vi "Lab Panel V4.87.vi"() -> ()   [LabVIEW 2013] (continued)
                                n557 = Unbundle(w898) -> ("Tmp Live"=w900:dbl, "Tmp Neut"=w899:dbl)  [unwired: 3 out]
                                n558 = Bundle(cluster=w902, "TL"=w900, "TN"=w899) -> (w901:cluster{"TL":dbl, "TN":dbl})
                                n559 = local write "TEMP START LAB01-2"(w901) -> ()
                              }
                            }
                          }
                        }
                      }
                    }
                  }
                }
              }
              event "RUN LAB02-1": Value Change {
                n560 = event-data() -> ("NewVal"=w907:bool)  [unwired: 1 in, 5 out]
                n561 = local read "SIG LAB02-1"() -> (w903:T2)
                n562 = case shown="True" w907 {
                  tunnel: w913 -> [_ w950]
                  tunnel: w912 -> [_ w949]
                  tunnel: w910 -> [w915 w948]
                  tunnel: w911 -> [_ w947]
                  tunnel: w909 -> [_ w946]
                  tunnel: [w914 w945] -> w908
                  tunnel: w906 -> [_ w944]
                  tunnel: w905 -> [_ w943]
                  tunnel: w904 -> [_ w942]
                  tunnel: w903 -> [_ w941]
                  frame False {
                    # "stop test"
                    n563 = stacked-sequence {
                      tunnel: w915 -> [w924 _]
                      tunnel: [w916 _] -> w914
                      frame #0 {
                        n564 = local read "DISP LAB02-1"() -> (w923:T4)
                        n565 = Unbundle(w923) -> ("CYCLE"=w921:dbl, "MINS"=w922:dbl)  [unwired: 1 out]
                        n566 = case shown="\"CYCLE TEST\"" w924 {
                          tunnel: w922 -> [_ _ w931]
                          tunnel: w921 -> [w929 w930 _]
                          tunnel: [w929 w930 w931] -> w920
                          frame "CHART TEST", Default {
                          }
                          frame "CYCLE TEST" {
                          }
                          frame "T-RISE TEST" {
                          }
                        }
                        n567 = local read "TDMS LAB02-1"() -> (w928:refnum<k34>)
                        n568 = Build Array("STOPPED") -> (w925:string[])
                        n569 = Build Array(w920) -> (w919:dbl[])
                        n570 = TDMS Write(0:w928, 5:"TEST RESULT", 7:w925, 9:w919) -> (4:w917:refnum<k34>, 15:w918:errorcluster)  [unwired: 2 in, 2 out]
                        n571 = TDMS Close(8:w918, 11:w917) -> (0:w916:errorcluster)  [unwired: 1 out]
                      }
                      frame #1 {
                        n572 = local read "DISP LAB02-1"() -> (w935:T4)
                        n573 = stacked-sequence {
                          tunnel: "LAB02-1" -> [w937 w939]
                          frame #0 {
                            n574 = call "sub vi - defrag tdms v1.vi"("panel id"=w937) -> ("error out"=w936:errorcluster)  [unwired: 10 in]
                            n575 = local write "data file error"(w936) -> ()
                          }
                          frame #1 {
                            n576 = local write "RESULT LAB02-1"(FALSE) -> ()
                            n577 = call "Save data file to network drive v2.vi"("panel id"=w939) -> ("network file save error"=w938:errorcluster)  [unwired: 9 in, 1 out]
                            n578 = local write "data file error"(w938) -> ()
                          }
                        }
                        n579 = Bundle(cluster=w935, "STATUS"="STOP") -> (w933:T4)  [unwired: 2 in]
                        n580 = local write "DISP LAB02-1"(w933) -> ()
                      }
                    }
                  }
                  frame True {
                    n581 = stacked-sequence {
                      seq-local: [w952 _] -> [_ w955]
                      tunnel: w950 -> [_ w965]
                      tunnel: w949 -> [_ w964]
                      tunnel: w948 -> [_ w963]
                      tunnel: w947 -> [_ w962]
                      tunnel: w946 -> [_ w961]
                      tunnel: [_ w960] -> w945
                      tunnel: w944 -> [_ w959]
                      tunnel: w943 -> [_ w958]
                      tunnel: w942 -> [_ w957]
                      tunnel: w941 -> [w951 w956]
                      frame #0 {
                        n582 = Unbundle(w951) -> ("AMPS"=w954:dbl)  [unwired: 4 out]
                        n583 = call "Check For Amps on v1.vi"("ID"="LAB02-1", "amps"=w954) -> ("amps"=w952:bool)  [unwired: 9 in]
                      }
                      frame #1 {
                        n584 = case shown="True" w955 {
                          tunnel: w965 -> [_ w977]
                          tunnel: w964 -> [_ w976]
                          tunnel: w963 -> [_ w975]
                          tunnel: w962 -> [_ w974]
                          tunnel: w961 -> [_ w973]
                          tunnel: [errorcluster {"status"=FALSE, "code"=0, "source"=""} ("error out") w972] -> w960
                          tunnel: w959 -> [_ w971]
                          tunnel: w958 -> [_ w970]
                          tunnel: w957 -> [_ w969]
                          tunnel: w956 -> [_ w968]
                          frame False {
                            w967 = FALSE
                            n585 = local write "RUN LAB02-1"(w967) -> ()
                            n586 = local write "run lab02-1"(w967) -> ()
                          }
                          frame True {
                            n587 = stacked-sequence {
                              seq-local: [w978 _ _ _ _] -> [_ w1002 _ _ _]
                              tunnel: w977 -> [w983 _ _ _ _]
                              tunnel: w976 -> [w980 _ _ _ _]
                              tunnel: w975 -> [w993 _ _ _ _]
                              tunnel: w974 -> [w986 _ _ _ _]
                              tunnel: w973 -> [w981 _ _ _ _]
                              tunnel: [_ w997 _ _ _] -> w972
                              tunnel: w971 -> [_ _ _ w1023 _]
                              tunnel: w970 -> [_ _ _ w1022 _]
                              tunnel: w969 -> [_ _ _ w1021 _]
                              tunnel: w968 -> [_ _ _ _ w1037]
                              frame #0 {
                                w979 = "\\"
                                n588 = local read "SET LAB02-1"() -> (w988:T5)
                                n589 = case shown="\"CYCLE TEST\"" w993 {
                                tunnel: ["L02-1-CHART TEST-" "L02-1-CYCLE TEST-" "L02-1-T-RISE TEST-"] -> w989
                                frame "CHART TEST", Default {
                                }
                                frame "CYCLE TEST" {
                                }
                                frame "T-RISE TEST" {
                                }
                                }
                                n590 = Unbundle(w988) -> ("DESCRIPTION"=w987:string)  [unwired: 4 out]
                                n591 = Concatenate Strings(w983, "\\", w981, w979, w980, w979) -> (w990:string)
                                n592 = String To Path(string=w990) -> (path=w992:path)
                                n593 = Concatenate Strings(w990, w989, w987, "-", w986, ".tdms") -> (w978:string)
                                n594 = Create Folder(path (use dialog)=w992) -> (error out=w991:errorcluster)  [unwired: 2 in, 2 out]
                                n595 = global write "Global 1.vi" "LAB02-1 FILE"(w978) -> ()
                                n596 = call <vilib>:"Clear Errors.vi"("error in (no error)"=w991) -> ()  [unwired: 6 in, 1 out]
                              }
                              frame #1 {
                                (unwired) FALSE
                                n597 = String To Path(string=w1002) -> (path=w998:path)
                                n598 = TDMS Open(6:FALSE, 10:T20."create or replace" ("operation (0:open)"), 11:w998) -> (0:w997:errorcluster, 3:→"TDMS LAB02-1":refnum<k34>)  [unwired: 4 in]
                              }
                              frame #2 {
                                n599 = local read "SET LAB02-1"() -> (w1008:T5)
                                n600 = local read "TDMS LAB02-1"() -> (w1019:refnum<k34>)
                                n601 = Build Array("Testers Name", "Description", "Set Test Cycles", "T-Rise minutes", "T-Rise Deg C") -> (w1009:string[])
                                n602 = Unbundle(w1008) -> ("NAME"=w1007:string, "DESCRIPTION"=w1006:string, "CYCLES"=w1005:dbl, "T-RISE mins"=w1004:dbl, "T-RISE deg C"=w1003:dbl)
                                n603 = Number To Decimal String(number=w1005) -> (decimal integer string=w1018:string)  [unwired: 1 in]
                                n604 = Number To Decimal String(number=w1004) -> (decimal integer string=w1017:string)  [unwired: 1 in]
                                n605 = Number To Decimal String(number=w1003) -> (decimal integer string=w1016:string)  [unwired: 1 in]
                                n606 = Build Array(w1007, w1006, w1018, w1017, w1016) -> (w1015:string[])
                                n607 = TDMS Set Properties(5:w1015, 7:w1009, 11:w1019) -> ()  [unwired: 3 in, 4 out]
                              }
                              frame #3 {
                                n608 = local read "DISP LAB02-1"() -> (w1024:T4)
                                n609 = Concatenate Strings("LAB02-1  ", w1023) -> (w1025:string)
                                n610 = Two Button Dialog(message=w1025, 1:w1021, 2:w1022) -> (T button?=w1027:bool)
                                n611 = case shown="True" w1027 {
                                tunnel: w1024 -> [w1034 w1035]
                                tunnel: [w1034 w1035] -> w1031
                                tunnel: [w1033 w1036] -> w1030
                                tunnel: [w1032 w1036] -> w1029
                                frame False {
                                n612 = Unbundle(w1034) -> ("CYCLE"=w1033:dbl, "MINS"=w1032:dbl)  [unwired: 1 out]
                                }
                                frame True {
                                w1036 = 0.0
                                }
                                }
                                n613 = Bundle(cluster=w1031, "CYCLE"=w1030, "MINS"=w1029, "STATUS"="RUN") -> (w1020:T4)
                                n614 = local write "DISP LAB02-1"(w1020) -> ()
                              }
                              frame #4 {
                                n615 = local read "TEMP START LAB02-1"() -> (w1041:cluster{"TL":dbl, "TN":dbl})
                                n616 = Unbundle(w1037) -> ("Tmp Live"=w1039:dbl, "Tmp Neut"=w1038:dbl)  [unwired: 3 out]
                                n617 = Bundle(cluster=w1041, "TL"=w1039, "TN"=w1038) -> (w1040:cluster{"TL":dbl, "TN":dbl})
                                n618 = local write "TEMP START LAB02-1"(w1040) -> ()
                              }
                            }
                          }
                        }
                      }
                    }
                  }
                }
                n619 = local write "run lab02-1"(w907) -> ()
              }
              event "RUN LAB02-2": Value Change {
                n620 = event-data() -> ("NewVal"=w1045:bool)  [unwired: 1 in, 5 out]
                n621 = local write "run lab02-2"(w1045) -> ()
                n622 = case shown="True" w1045 {
                  tunnel: w1051 -> [_ w1088]
                  tunnel: w1050 -> [_ w1087]
                  tunnel: w1048 -> [w1053 w1086]
                  tunnel: w1049 -> [_ w1085]
                  tunnel: w1047 -> [_ w1084]
                  tunnel: [w1052 w1083] -> w1046
                  tunnel: w1044 -> [_ w1082]
                  tunnel: w1043 -> [_ w1081]
                  tunnel: w1042 -> [_ w1080]
                  frame False {
                    # "stop test"
                    n623 = stacked-sequence {
                      tunnel: w1053 -> [w1062 _]
                      tunnel: [w1054 _] -> w1052
                      frame #0 {
                        n624 = local read "DISP LAB02-2"() -> (w1061:T4)
                        n625 = Unbundle(w1061) -> ("CYCLE"=w1059:dbl, "MINS"=w1060:dbl)  [unwired: 1 out]
                        n626 = case shown="\"CYCLE TEST\"" w1062 {
                          tunnel: w1060 -> [_ _ w1069]
                          tunnel: w1059 -> [w1067 w1068 _]
                          tunnel: [w1067 w1068 w1069] -> w1058
                          frame "CHART TEST", Default {
                          }
                          frame "CYCLE TEST" {
                          }
                          frame "T-RISE TEST" {
                          }
                        }
                        n627 = local read "TDMS LAB02-2"() -> (w1066:refnum<k34>)
                        n628 = Build Array("STOPPED") -> (w1063:string[])
                        n629 = Build Array(w1058) -> (w1057:dbl[])
                        n630 = TDMS Write(0:w1066, 5:"TEST RESULT", 7:w1063, 9:w1057) -> (4:w1055:refnum<k34>, 15:w1056:errorcluster)  [unwired: 2 in, 2 out]
                        n631 = TDMS Close(8:w1056, 11:w1055) -> (0:w1054:errorcluster)  [unwired: 1 out]
                      }
                      frame #1 {
                        n632 = local read "DISP LAB02-2"() -> (w1073:T4)
                        n633 = stacked-sequence {
                          tunnel: "LAB02-2" -> [w1075 w1077]
                          frame #0 {
                            n634 = call "sub vi - defrag tdms v1.vi"("panel id"=w1075) -> ("error out"=w1074:errorcluster)  [unwired: 10 in]
                            n635 = local write "data file error"(w1074) -> ()
                          }
                          frame #1 {
                            n636 = call "Save data file to network drive v2.vi"("panel id"=w1077) -> ("network file save error"=w1076:errorcluster)  [unwired: 9 in, 1 out]
                            n637 = local write "RESULT LAB02-2"(FALSE) -> ()
                            n638 = local write "data file error"(w1076) -> ()
                          }
                        }
                        n639 = Bundle(cluster=w1073, "STATUS"="STOP") -> (w1071:T4)  [unwired: 2 in]
                        n640 = local write "DISP LAB02-2"(w1071) -> ()
                      }
                    }
                  }
                  frame True {
                    n641 = local read "SIG LAB02-2"() -> (w1079:T2)
                    n642 = stacked-sequence {
                      seq-local: [w1090 _] -> [_ w1093]
                      tunnel: w1088 -> [_ w1103]
                      tunnel: w1087 -> [_ w1102]
                      tunnel: w1086 -> [_ w1101]
                      tunnel: w1085 -> [_ w1100]
                      tunnel: w1084 -> [_ w1099]
                      tunnel: [_ w1098] -> w1083
                      tunnel: w1082 -> [_ w1097]
                      tunnel: w1081 -> [_ w1096]
                      tunnel: w1080 -> [_ w1095]
                      tunnel: w1079 -> [w1089 w1094]
                      frame #0 {
                        n643 = Unbundle(w1089) -> ("AMPS"=w1092:dbl)  [unwired: 4 out]
                        n644 = call "Check For Amps on v1.vi"("ID"="LAB02-2", "amps"=w1092) -> ("amps"=w1090:bool)  [unwired: 9 in]
                      }
                      frame #1 {
                        n645 = case shown="True" w1093 {
                          tunnel: w1103 -> [_ w1115]
                          tunnel: w1102 -> [_ w1114]
                          tunnel: w1101 -> [_ w1113]
                          tunnel: w1100 -> [_ w1112]
                          tunnel: w1099 -> [_ w1111]
                          tunnel: [errorcluster {"status"=FALSE, "code"=0, "source"=""} ("error out") w1110] -> w1098
                          tunnel: w1097 -> [_ w1109]
                          tunnel: w1096 -> [_ w1108]
                          tunnel: w1095 -> [_ w1107]
                          tunnel: w1094 -> [_ w1106]
                          frame False {
                            w1104 = FALSE
                            n646 = local write "RUN LAB02-2"(w1104) -> ()
                            n647 = local write "run lab02-2"(w1104) -> ()
                          }
                          frame True {
                            n648 = stacked-sequence {
                              seq-local: [w1116 _ _ _ _] -> [_ w1140 _ _ _]
                              tunnel: w1115 -> [w1121 _ _ _ _]
                              tunnel: w1114 -> [w1118 _ _ _ _]
                              tunnel: w1113 -> [w1131 _ _ _ _]
                              tunnel: w1112 -> [w1124 _ _ _ _]
                              tunnel: w1111 -> [w1119 _ _ _ _]
                              tunnel: [_ w1135 _ _ _] -> w1110
                              tunnel: w1109 -> [_ _ _ w1161 _]
                              tunnel: w1108 -> [_ _ _ w1160 _]
                              tunnel: w1107 -> [_ _ _ w1159 _]
                              tunnel: w1106 -> [_ _ _ _ w1175]
                              frame #0 {
                                w1117 = "\\"
                                n649 = local read "SET LAB02-2"() -> (w1126:T5)
                                n650 = case shown="\"CYCLE TEST\"" w1131 {
                                tunnel: ["L02-2-CHART TEST-" "L02-2-CYCLE TEST-" "L02-2-T-RISE TEST-"] -> w1127
                                frame "CHART TEST", Default {
                                }
                                frame "CYCLE TEST" {
                                }
                                frame "T-RISE TEST" {
                                }
                                }
                                n651 = Unbundle(w1126) -> ("DESCRIPTION"=w1125:string)  [unwired: 4 out]
                                n652 = Concatenate Strings(w1121, "\\", w1119, w1117, w1118, w1117) -> (w1128:string)
                                n653 = String To Path(string=w1128) -> (path=w1130:path)
                                n654 = Concatenate Strings(w1128, w1127, w1125, "-", w1124, ".tdms") -> (w1116:string)
                                n655 = Create Folder(path (use dialog)=w1130) -> (error out=w1129:errorcluster)  [unwired: 2 in, 2 out]
                                n656 = global write "Global 1.vi" "LAB02-2 FILE"(w1116) -> ()
                                n657 = call <vilib>:"Clear Errors.vi"("error in (no error)"=w1129) -> ()  [unwired: 6 in, 1 out]
                              }
                              frame #1 {
                                (unwired) FALSE
                                n658 = String To Path(string=w1140) -> (path=w1136:path)
                                n659 = TDMS Open(6:FALSE, 10:T20."create or replace" ("operation (0:open)"), 11:w1136) -> (0:w1135:errorcluster, 3:→"TDMS LAB02-2":refnum<k34>)  [unwired: 4 in]
                              }
                              frame #2 {
                                n660 = local read "SET LAB02-2"() -> (w1146:T5)
                                n661 = local read "TDMS LAB02-2"() -> (w1157:refnum<k34>)
                                n662 = Build Array("Testers Name", "Description", "Set Test Cycles", "T-Rise minutes", "T-Rise Deg C") -> (w1147:string[])
                                n663 = Unbundle(w1146) -> ("NAME"=w1145:string, "DESCRIPTION"=w1144:string, "CYCLES"=w1143:dbl, "T-RISE mins"=w1142:dbl, "T-RISE deg C"=w1141:dbl)
                                n664 = Number To Decimal String(number=w1143) -> (decimal integer string=w1156:string)  [unwired: 1 in]
                                n665 = Number To Decimal String(number=w1142) -> (decimal integer string=w1155:string)  [unwired: 1 in]
                                n666 = Number To Decimal String(number=w1141) -> (decimal integer string=w1154:string)  [unwired: 1 in]
                                n667 = Build Array(w1145, w1144, w1156, w1155, w1154) -> (w1153:string[])
                                n668 = TDMS Set Properties(5:w1153, 7:w1147, 11:w1157) -> ()  [unwired: 3 in, 4 out]
                              }
                              frame #3 {
                                n669 = local read "DISP LAB02-2"() -> (w1162:T4)
                                n670 = Concatenate Strings("LAB02-2  ", w1161) -> (w1163:string)
                                n671 = Two Button Dialog(message=w1163, 1:w1159, 2:w1160) -> (T button?=w1165:bool)
                                n672 = case shown="True" w1165 {
                                tunnel: w1162 -> [w1172 w1173]
                                tunnel: [w1172 w1173] -> w1169
                                tunnel: [w1171 w1174] -> w1168
                                tunnel: [w1170 w1174] -> w1167
                                frame False {
                                n673 = Unbundle(w1172) -> ("CYCLE"=w1171:dbl, "MINS"=w1170:dbl)  [unwired: 1 out]
                                }
                                frame True {
                                w1174 = 0.0
                                }
                                }
                                n674 = Bundle(cluster=w1169, "CYCLE"=w1168, "MINS"=w1167, "STATUS"="RUN") -> (w1158:T4)
                                n675 = local write "DISP LAB02-2"(w1158) -> ()
                              }
                              frame #4 {
                                n676 = local read "TEMP START LAB02-2"() -> (w1179:cluster{"TL":dbl, "TN":dbl})
                                n677 = Unbundle(w1175) -> ("Tmp Live"=w1177:dbl, "Tmp Neut"=w1176:dbl)  [unwired: 3 out]
                                n678 = Bundle(cluster=w1179, "TL"=w1177, "TN"=w1176) -> (w1178:cluster{"TL":dbl, "TN":dbl})
                                n679 = local write "TEMP START LAB02-2"(w1178) -> ()
                              }
                            }
                          }
                        }
                      }
                    }
                  }
                }
              }
              event "RUN LAB03-1": Value Change {
                n680 = event-data() -> ("NewVal"=w1183:bool)  [unwired: 1 in, 5 out]
                n681 = local write "run lab03-1"(w1183) -> ()
                n682 = case shown="True" w1183 {
                  tunnel: w1189 -> [_ w1226]
                  tunnel: w1188 -> [_ w1225]
                  tunnel: w1186 -> [w1191 w1224]
                  tunnel: w1187 -> [_ w1223]
                  tunnel: w1185 -> [_ w1222]
                  tunnel: [w1190 w1221] -> w1184
                  tunnel: w1182 -> [_ w1220]
                  tunnel: w1181 -> [_ w1219]
                  tunnel: w1180 -> [_ w1218]
                  frame False {
                    # "stop test"
                    n683 = stacked-sequence {
                      tunnel: w1191 -> [w1200 _]
                      tunnel: [w1192 _] -> w1190
                      frame #0 {
                        n684 = local read "DISP LAB03-1"() -> (w1199:T4)
                        n685 = Unbundle(w1199) -> ("CYCLE"=w1197:dbl, "MINS"=w1198:dbl)  [unwired: 1 out]
                        n686 = case shown="\"CYCLE TEST\"" w1200 {
                          tunnel: w1198 -> [_ _ w1207]
                          tunnel: w1197 -> [w1205 w1206 _]
                          tunnel: [w1205 w1206 w1207] -> w1196
                          frame "CHART TEST", Default {
                          }
                          frame "CYCLE TEST" {
                          }
                          frame "T-RISE TEST" {
                          }
                        }
                        n687 = local read "TDMS LAB03-1"() -> (w1204:refnum<k34>)
                        n688 = Build Array("STOPPED") -> (w1201:string[])
                        n689 = Build Array(w1196) -> (w1195:dbl[])
                        n690 = TDMS Write(0:w1204, 5:"TEST RESULT", 7:w1201, 9:w1195) -> (4:w1193:refnum<k34>, 15:w1194:errorcluster)  [unwired: 2 in, 2 out]
                        n691 = TDMS Close(8:w1194, 11:w1193) -> (0:w1192:errorcluster)  [unwired: 1 out]
                      }
                      frame #1 {
                        n692 = local read "DISP LAB03-1"() -> (w1211:T4)
                        n693 = stacked-sequence {
                          tunnel: "LAB03-1" -> [w1213 w1215]
                          frame #0 {
                            n694 = call "sub vi - defrag tdms v1.vi"("panel id"=w1213) -> ("error out"=w1212:errorcluster)  [unwired: 10 in]
                            n695 = local write "data file error"(w1212) -> ()
                          }
                          frame #1 {
                            n696 = call "Save data file to network drive v2.vi"("panel id"=w1215) -> ("network file save error"=w1214:errorcluster)  [unwired: 9 in, 1 out]
                            n697 = local write "RESULT LAB03-1"(FALSE) -> ()
                            n698 = local write "data file error"(w1214) -> ()
                          }
                        }
                        n699 = Bundle(cluster=w1211, "STATUS"="STOP") -> (w1209:T4)  [unwired: 2 in]
                        n700 = local write "DISP LAB03-1"(w1209) -> ()
                      }
                    }
                  }
                  frame True {
                    n701 = local read "SIG LAB03-1"() -> (w1217:T2)
                    n702 = stacked-sequence {
                      seq-local: [w1228 _] -> [_ w1231]
                      tunnel: w1226 -> [_ w1241]
                      tunnel: w1225 -> [_ w1240]
                      tunnel: w1224 -> [_ w1239]
                      tunnel: w1223 -> [_ w1238]
                      tunnel: w1222 -> [_ w1237]
                      tunnel: [_ w1236] -> w1221
                      tunnel: w1220 -> [_ w1235]
                      tunnel: w1219 -> [_ w1234]
                      tunnel: w1218 -> [_ w1233]
                      tunnel: w1217 -> [w1227 w1232]
                      frame #0 {
                        n703 = Unbundle(w1227) -> ("AMPS"=w1230:dbl)  [unwired: 4 out]
                        n704 = call "Check For Amps on v1.vi"("ID"="LAB03-1", "amps"=w1230) -> ("amps"=w1228:bool)  [unwired: 9 in]
                      }
                      frame #1 {
                        n705 = case shown="True" w1231 {
                          tunnel: w1241 -> [_ w1253]
                          tunnel: w1240 -> [_ w1252]
                          tunnel: w1239 -> [_ w1251]
                          tunnel: w1238 -> [_ w1250]
                          tunnel: w1237 -> [_ w1249]
                          tunnel: [errorcluster {"status"=FALSE, "code"=0, "source"=""} ("error out") w1248] -> w1236
                          tunnel: w1235 -> [_ w1247]
                          tunnel: w1234 -> [_ w1246]
                          tunnel: w1233 -> [_ w1245]
                          tunnel: w1232 -> [_ w1244]
                          frame False {
                            w1242 = FALSE
                            n706 = local write "RUN LAB03-1"(w1242) -> ()
                            n707 = local write "run lab03-1"(w1242) -> ()
                          }
                          frame True {
                            n708 = stacked-sequence {
                              seq-local: [w1254 _ _ _ _] -> [_ w1278 _ _ _]
                              tunnel: w1253 -> [w1259 _ _ _ _]
                              tunnel: w1252 -> [w1256 _ _ _ _]
                              tunnel: w1251 -> [w1269 _ _ _ _]
                              tunnel: w1250 -> [w1262 _ _ _ _]
                              tunnel: w1249 -> [w1257 _ _ _ _]
                              tunnel: [_ w1273 _ _ _] -> w1248
                              tunnel: w1247 -> [_ _ _ w1298 _]
                              tunnel: w1246 -> [_ _ _ w1297 _]
                              tunnel: w1245 -> [_ _ _ w1296 _]
                              tunnel: w1244 -> [_ _ _ _ w1313]
                              frame #0 {
                                w1255 = "\\"
                                n709 = local read "SET LAB03-1"() -> (w1264:T5)
                                n710 = case shown="\"T-RISE TEST\"" w1269 {
                                tunnel: ["L03-1-CHART TEST-" "L03-1-CYCLE TEST-" "L03-1-T-RISE TEST-"] -> w1265
                                frame "CHART TEST", Default {
                                }
                                frame "CYCLE TEST" {
                                }
                                frame "T-RISE TEST" {
                                }
                                }
                                n711 = Unbundle(w1264) -> ("DESCRIPTION"=w1263:string)  [unwired: 4 out]
                                n712 = Concatenate Strings(w1259, "\\", w1257, w1255, w1256, w1255) -> (w1266:string)
                                n713 = String To Path(string=w1266) -> (path=w1268:path)
                                n714 = Concatenate Strings(w1266, w1265, w1263, "-", w1262, ".tdms") -> (w1254:string)
                                n715 = Create Folder(path (use dialog)=w1268) -> (error out=w1267:errorcluster)  [unwired: 2 in, 2 out]
                                n716 = global write "Global 1.vi" "LAB03-1 FILE"(w1254) -> ()
                                n717 = call <vilib>:"Clear Errors.vi"("error in (no error)"=w1267) -> ()  [unwired: 6 in, 1 out]
                              }
                              frame #1 {
                                (unwired) FALSE
                                n718 = String To Path(string=w1278) -> (path=w1274:path)
                                n719 = TDMS Open(6:FALSE, 10:T20."create or replace" ("operation (0:open)"), 11:w1274) -> (0:w1273:errorcluster, 3:→"TDMS LAB03-1":refnum<k34>)  [unwired: 4 in]
                              }
                              frame #2 {
                                n720 = local read "SET LAB03-1"() -> (w1284:T5)
                                n721 = local read "TDMS LAB03-1"() -> (w1295:refnum<k34>)
                                n722 = Build Array("Testers Name", "Description", "Set Test Cycles", "T-Rise minutes", "T-Rise Deg C") -> (w1285:string[])
                                n723 = Unbundle(w1284) -> ("NAME"=w1283:string, "DESCRIPTION"=w1282:string, "CYCLES"=w1281:dbl, "T-RISE mins"=w1280:dbl, "T-RISE deg C"=w1279:dbl)
                                n724 = Number To Decimal String(number=w1281) -> (decimal integer string=w1294:string)  [unwired: 1 in]
                                n725 = Number To Decimal String(number=w1280) -> (decimal integer string=w1293:string)  [unwired: 1 in]
                                n726 = Number To Decimal String(number=w1279) -> (decimal integer string=w1292:string)  [unwired: 1 in]
                                n727 = Build Array(w1283, w1282, w1294, w1293, w1292) -> (w1291:string[])
                                n728 = TDMS Set Properties(5:w1291, 7:w1285, 11:w1295) -> ()  [unwired: 3 in, 4 out]
                              }
                              frame #3 {
                                n729 = local read "DISP LAB03-1"() -> (w1300:T4)
                                n730 = Concatenate Strings("LAB03-1  ", w1298) -> (w1301:string)
                                n731 = Two Button Dialog(message=w1301, 1:w1296, 2:w1297) -> (T button?=w1303:bool)
                                n732 = case shown="True" w1303 {
                                tunnel: w1300 -> [w1310 w1311]
                                tunnel: [w1310 w1311] -> w1307
                                tunnel: [w1309 w1312] -> w1306
                                tunnel: [w1308 w1312] -> w1305
                                frame False {
                                n733 = Unbundle(w1310) -> ("CYCLE"=w1309:dbl, "MINS"=w1308:dbl)  [unwired: 1 out]
                                }
                                frame True {
                                w1312 = 0.0
                                }
                                }
                                n734 = Bundle(cluster=w1307, "CYCLE"=w1306, "MINS"=w1305, "STATUS"="RUN") -> (w1299:T4)
                                n735 = local write "DISP LAB03-1"(w1299) -> ()
                              }
                              frame #4 {
                                n736 = local read "TEMP START LAB03-1"() -> (w1317:cluster{"TL":dbl, "TN":dbl})
                                n737 = Unbundle(w1313) -> ("Tmp Live"=w1315:dbl, "Tmp Neut"=w1314:dbl)  [unwired: 3 out]
                                n738 = Bundle(cluster=w1317, "TL"=w1315, "TN"=w1314) -> (w1316:cluster{"TL":dbl, "TN":dbl})
                                n739 = local write "TEMP START LAB03-1"(w1316) -> ()
                              }
                            }
                          }
                        }
                      }
                    }
                  }
                }
              }
              event "RUN LAB03-2": Value Change {
                n740 = event-data() -> ("NewVal"=w1321:bool)  [unwired: 1 in, 5 out]
                n741 = local write "run lab03-2"(w1321) -> ()
                n742 = case shown="True" w1321 {
                  tunnel: w1327 -> [_ w1364]
                  tunnel: w1326 -> [_ w1363]
                  tunnel: w1324 -> [w1329 w1362]
                  tunnel: w1325 -> [_ w1361]
                  tunnel: w1323 -> [_ w1360]
                  tunnel: [w1328 w1359] -> w1322
                  tunnel: w1320 -> [_ w1358]
                  tunnel: w1319 -> [_ w1357]
                  tunnel: w1318 -> [_ w1356]
                  frame False {
                    # "stop test"
                    n743 = stacked-sequence {
                      tunnel: w1329 -> [w1338 _]
                      tunnel: [w1330 _] -> w1328
                      frame #0 {
                        n744 = local read "DISP LAB03-2"() -> (w1337:T4)
                        n745 = Unbundle(w1337) -> ("CYCLE"=w1335:dbl, "MINS"=w1336:dbl)  [unwired: 1 out]
                        n746 = case shown="\"CYCLE TEST\"" w1338 {
                          tunnel: w1336 -> [_ _ w1345]
                          tunnel: w1335 -> [w1343 w1344 _]
                          tunnel: [w1343 w1344 w1345] -> w1334
                          frame "CHART TEST", Default {
                          }
                          frame "CYCLE TEST" {
                          }
                          frame "T-RISE TEST" {
                          }
                        }
                        n747 = local read "TDMS LAB03-2"() -> (w1342:refnum<k34>)
                        n748 = Build Array("STOPPED") -> (w1339:string[])
                        n749 = Build Array(w1334) -> (w1333:dbl[])
                        n750 = TDMS Write(0:w1342, 5:"TEST RESULT", 7:w1339, 9:w1333) -> (4:w1331:refnum<k34>, 15:w1332:errorcluster)  [unwired: 2 in, 2 out]
                        n751 = TDMS Close(8:w1332, 11:w1331) -> (0:w1330:errorcluster)  [unwired: 1 out]
                      }
                      frame #1 {
                        n752 = local read "DISP LAB03-2"() -> (w1349:T4)
                        n753 = stacked-sequence {
                          tunnel: "LAB03-2" -> [w1351 w1353]
                          frame #0 {
                            n754 = call "sub vi - defrag tdms v1.vi"("panel id"=w1351) -> ("error out"=w1350:errorcluster)  [unwired: 10 in]
                            n755 = local write "data file error"(w1350) -> ()
                          }
                          frame #1 {
                            n756 = call "Save data file to network drive v2.vi"("panel id"=w1353) -> ("network file save error"=w1352:errorcluster)  [unwired: 9 in, 1 out]
                            n757 = local write "RESULT LAB03-2"(FALSE) -> ()
                            n758 = local write "data file error"(w1352) -> ()
                          }
                        }
                        n759 = Bundle(cluster=w1349, "STATUS"="STOP") -> (w1347:T4)  [unwired: 2 in]
                        n760 = local write "DISP LAB03-2"(w1347) -> ()
                      }
                    }
                  }
                  frame True {
                    n761 = local read "SIG LAB03-2"() -> (w1355:T2)
                    n762 = stacked-sequence {
                      seq-local: [w1366 _] -> [_ w1369]
                      tunnel: w1364 -> [_ w1379]
                      tunnel: w1363 -> [_ w1378]
                      tunnel: w1362 -> [_ w1377]
                      tunnel: w1361 -> [_ w1376]
                      tunnel: w1360 -> [_ w1375]
                      tunnel: [_ w1374] -> w1359
                      tunnel: w1358 -> [_ w1373]
                      tunnel: w1357 -> [_ w1372]
                      tunnel: w1356 -> [_ w1371]
                      tunnel: w1355 -> [w1365 w1370]
                      frame #0 {
                        n763 = Unbundle(w1365) -> ("AMPS"=w1368:dbl)  [unwired: 4 out]
                        n764 = call "Check For Amps on v1.vi"("ID"="LAB03-2", "amps"=w1368) -> ("amps"=w1366:bool)  [unwired: 9 in]
                      }
                      frame #1 {
                        n765 = case shown="True" w1369 {
                          tunnel: w1379 -> [_ w1391]
                          tunnel: w1378 -> [_ w1390]
                          tunnel: w1377 -> [_ w1389]
                          tunnel: w1376 -> [_ w1388]
                          tunnel: w1375 -> [_ w1387]
                          tunnel: [errorcluster {"status"=FALSE, "code"=0, "source"=""} ("error out") w1386] -> w1374
                          tunnel: w1373 -> [_ w1385]
                          tunnel: w1372 -> [_ w1384]
                          tunnel: w1371 -> [_ w1383]
                          tunnel: w1370 -> [_ w1382]
                          frame False {
                            w1380 = FALSE
                            n766 = local write "RUN LAB03-2"(w1380) -> ()
                            n767 = local write "run lab03-2"(w1380) -> ()
                          }
                          frame True {
                            n768 = stacked-sequence {
                              seq-local: [w1392 _ _ _ _] -> [_ w1416 _ _ _]
                              tunnel: w1391 -> [w1397 _ _ _ _]
                              tunnel: w1390 -> [w1394 _ _ _ _]
                              tunnel: w1389 -> [w1407 _ _ _ _]
                              tunnel: w1388 -> [w1400 _ _ _ _]
                              tunnel: w1387 -> [w1395 _ _ _ _]
                              tunnel: [_ w1411 _ _ _] -> w1386
                              tunnel: w1385 -> [_ _ _ w1437 _]
                              tunnel: w1384 -> [_ _ _ w1436 _]
                              tunnel: w1383 -> [_ _ _ w1435 _]
                              tunnel: w1382 -> [_ _ _ _ w1451]
                              frame #0 {
                                w1393 = "\\"
                                n769 = local read "SET LAB03-2"() -> (w1402:T5)
                                n770 = case shown="\"T-RISE TEST\"" w1407 {
                                tunnel: ["L03-2-CHART TEST-" "L03-2-CYCLE TEST-" "L03-2-T-RISE TEST-"] -> w1403
                                frame "CHART TEST", Default {
                                }
                                frame "CYCLE TEST" {
                                }
                                frame "T-RISE TEST" {
                                }
                                }
                                n771 = Unbundle(w1402) -> ("DESCRIPTION"=w1401:string)  [unwired: 4 out]
                                n772 = Concatenate Strings(w1397, "\\", w1395, w1393, w1394, w1393) -> (w1404:string)
                                n773 = String To Path(string=w1404) -> (path=w1406:path)
                                n774 = Concatenate Strings(w1404, w1403, w1401, "-", w1400, ".tdms") -> (w1392:string)
                                n775 = Create Folder(path (use dialog)=w1406) -> (error out=w1405:errorcluster)  [unwired: 2 in, 2 out]
                                n776 = global write "Global 1.vi" "LAB03-2 FILE"(w1392) -> ()
                                n777 = call <vilib>:"Clear Errors.vi"("error in (no error)"=w1405) -> ()  [unwired: 6 in, 1 out]
                              }
                              frame #1 {
                                (unwired) FALSE
                                n778 = String To Path(string=w1416) -> (path=w1412:path)
                                n779 = TDMS Open(6:FALSE, 10:T20."create or replace" ("operation (0:open)"), 11:w1412) -> (0:w1411:errorcluster, 3:→"TDMS LAB03-2":refnum<k34>)  [unwired: 4 in]
                              }
                              frame #2 {
                                n780 = local read "SET LAB03-2"() -> (w1422:T5)
                                n781 = local read "TDMS LAB03-2"() -> (w1433:refnum<k34>)
                                n782 = Build Array("Testers Name", "Description", "Set Test Cycles", "T-Rise minutes", "T-Rise Deg C") -> (w1423:string[])
                                n783 = Unbundle(w1422) -> ("NAME"=w1421:string, "DESCRIPTION"=w1420:string, "CYCLES"=w1419:dbl, "T-RISE mins"=w1418:dbl, "T-RISE deg C"=w1417:dbl)
                                n784 = Number To Decimal String(number=w1419) -> (decimal integer string=w1432:string)  [unwired: 1 in]
                                n785 = Number To Decimal String(number=w1418) -> (decimal integer string=w1431:string)  [unwired: 1 in]
                                n786 = Number To Decimal String(number=w1417) -> (decimal integer string=w1430:string)  [unwired: 1 in]
                                n787 = Build Array(w1421, w1420, w1432, w1431, w1430) -> (w1429:string[])
                                n788 = TDMS Set Properties(5:w1429, 7:w1423, 11:w1433) -> ()  [unwired: 3 in, 4 out]
                              }
                              frame #3 {
                                n789 = local read "DISP LAB03-2"() -> (w1438:T4)
                                n790 = Concatenate Strings("LAB03-2  ", w1437) -> (w1439:string)
                                n791 = Two Button Dialog(message=w1439, 1:w1435, 2:w1436) -> (T button?=w1441:bool)
                                n792 = case shown="True" w1441 {
                                tunnel: w1438 -> [w1448 w1449]
                                tunnel: [w1448 w1449] -> w1445
                                tunnel: [w1447 w1450] -> w1444
                                tunnel: [w1446 w1450] -> w1443
                                frame False {
                                n793 = Unbundle(w1448) -> ("CYCLE"=w1447:dbl, "MINS"=w1446:dbl)  [unwired: 1 out]
                                }
                                frame True {
                                w1450 = 0.0
                                }
                                }
                                n794 = Bundle(cluster=w1445, "CYCLE"=w1444, "MINS"=w1443, "STATUS"="RUN") -> (w1434:T4)
                                n795 = local write "DISP LAB03-2"(w1434) -> ()
                              }
                              frame #4 {
                                n796 = local read "TEMP START LAB03-2"() -> (w1455:cluster{"TL":dbl, "TN":dbl})
                                n797 = Unbundle(w1451) -> ("Tmp Live"=w1453:dbl, "Tmp Neut"=w1452:dbl)  [unwired: 3 out]
                                n798 = Bundle(cluster=w1455, "TL"=w1453, "TN"=w1452) -> (w1454:cluster{"TL":dbl, "TN":dbl})
                                n799 = local write "TEMP START LAB03-2"(w1454) -> ()
                              }
                            }
                          }
                        }
                      }
                    }
                  }
                }
              }
              event "RUN LAB04-1": Value Change {
                n800 = event-data() -> ("NewVal"=w1459:bool)  [unwired: 1 in, 5 out]
                n801 = local write "run lab04-1"(w1459) -> ()
                n802 = case shown="True" w1459 {
                  tunnel: w1465 -> [_ w1502]
                  tunnel: w1464 -> [_ w1501]
                  tunnel: w1462 -> [w1467 w1500]
                  tunnel: w1463 -> [_ w1499]
                  tunnel: w1461 -> [_ w1498]
                  tunnel: [w1466 w1497] -> w1460
                  tunnel: w1458 -> [_ w1496]
                  tunnel: w1457 -> [_ w1495]
                  tunnel: w1456 -> [_ w1494]
                  frame False {
                    # "stop test"
                    n803 = stacked-sequence {
                      tunnel: w1467 -> [w1476 _]
                      tunnel: [w1468 _] -> w1466
                      frame #0 {
                        n804 = local read "DISP LAB04-1"() -> (w1475:T4)
                        n805 = Unbundle(w1475) -> ("CYCLE"=w1473:dbl, "MINS"=w1474:dbl)  [unwired: 1 out]
                        n806 = case shown="\"CYCLE TEST\"" w1476 {
                          tunnel: w1474 -> [_ _ w1483]
                          tunnel: w1473 -> [w1481 w1482 _]
                          tunnel: [w1481 w1482 w1483] -> w1472
                          frame "CHART TEST", Default {
                          }
                          frame "CYCLE TEST" {
                          }
                          frame "T-RISE TEST" {
                          }
                        }
                        n807 = local read "TDMS LAB04-1"() -> (w1480:refnum<k34>)
                        n808 = Build Array("STOPPED") -> (w1477:string[])
                        n809 = Build Array(w1472) -> (w1471:dbl[])
                        n810 = TDMS Write(0:w1480, 5:"TEST RESULT", 7:w1477, 9:w1471) -> (4:w1469:refnum<k34>, 15:w1470:errorcluster)  [unwired: 2 in, 2 out]
                        n811 = TDMS Close(8:w1470, 11:w1469) -> (0:w1468:errorcluster)  [unwired: 1 out]
                      }
                      frame #1 {
                        n812 = local read "DISP LAB04-1"() -> (w1487:T4)
                        n813 = stacked-sequence {
                          tunnel: "LAB04-1" -> [w1489 w1491]
                          frame #0 {
                            n814 = call "sub vi - defrag tdms v1.vi"("panel id"=w1489) -> ("error out"=w1488:errorcluster)  [unwired: 10 in]
                            n815 = local write "data file error"(w1488) -> ()
                          }
                          frame #1 {
                            n816 = call "Save data file to network drive v2.vi"("panel id"=w1491) -> ("network file save error"=w1490:errorcluster)  [unwired: 9 in, 1 out]
                            n817 = local write "RESULT LAB04-1"(FALSE) -> ()
                            n818 = local write "data file error"(w1490) -> ()
                          }
                        }
                        n819 = Bundle(cluster=w1487, "STATUS"="STOP") -> (w1485:T4)  [unwired: 2 in]
                        n820 = local write "DISP LAB04-1"(w1485) -> ()
                      }
                    }
                  }
                  frame True {
                    n821 = local read "SIG LAB04-1"() -> (w1493:T2)
                    n822 = stacked-sequence {
                      seq-local: [w1504 _] -> [_ w1507]
                      tunnel: w1502 -> [_ w1517]
                      tunnel: w1501 -> [_ w1516]
                      tunnel: w1500 -> [_ w1515]
                      tunnel: w1499 -> [_ w1514]
                      tunnel: w1498 -> [_ w1513]
                      tunnel: [_ w1512] -> w1497
                      tunnel: w1496 -> [_ w1511]
                      tunnel: w1495 -> [_ w1510]
                      tunnel: w1494 -> [_ w1509]
                      tunnel: w1493 -> [w1503 w1508]
                      frame #0 {
                        n823 = Unbundle(w1503) -> ("AMPS"=w1506:dbl)  [unwired: 4 out]
                        n824 = call "Check For Amps on v1.vi"("ID"="LAB04-1", "amps"=w1506) -> ("amps"=w1504:bool)  [unwired: 9 in]
                      }
                      frame #1 {
                        n825 = case shown="True" w1507 {
                          tunnel: w1517 -> [_ w1529]
                          tunnel: w1516 -> [_ w1528]
                          tunnel: w1515 -> [_ w1527]
                          tunnel: w1514 -> [_ w1526]
                          tunnel: w1513 -> [_ w1525]
                          tunnel: [errorcluster {"status"=FALSE, "code"=0, "source"=""} ("error out") w1524] -> w1512
                          tunnel: w1511 -> [_ w1523]
                          tunnel: w1510 -> [_ w1522]
                          tunnel: w1509 -> [_ w1521]
                          tunnel: w1508 -> [_ w1520]
                          frame False {
                            w1518 = FALSE
                            n826 = local write "RUN LAB04-1"(w1518) -> ()
                            n827 = local write "run lab04-1"(w1518) -> ()
                          }
                          frame True {
                            n828 = stacked-sequence {
                              seq-local: [w1530 _ _ _ _] -> [_ w1554 _ _ _]
                              tunnel: w1529 -> [w1535 _ _ _ _]
                              tunnel: w1528 -> [w1531 _ _ _ _]
                              tunnel: w1527 -> [w1545 _ _ _ _]
                              tunnel: w1526 -> [w1538 _ _ _ _]
                              tunnel: w1525 -> [w1533 _ _ _ _]
                              tunnel: [_ w1549 _ _ _] -> w1524
                              tunnel: w1523 -> [_ _ _ w1575 _]
                              tunnel: w1522 -> [_ _ _ w1574 _]
                              tunnel: w1521 -> [_ _ _ w1573 _]
                              tunnel: w1520 -> [_ _ _ _ w1589]
                              frame #0 {
                                w1532 = "\\"
